vi "example_2_2010.vi"() -> ()   [LabVIEW 2010]
uses:
  <vilib>/Analysis/NI_AALBase.lvlib
  <vilib>/Analysis/baseanly.llb/Mean (DBL).vi
panel:
  out "Time with \"On\"":u32
  out "Time with \"Auto\"":u32
  in  "Time dimensions":bool
  out "MAE Theil-Sen (Off)":dbl format="%0.2f"
  out "MAE Theil-Sen (Auto)":dbl format="%0.2f"
  out "XY Graph":cluster{dbl[], dbl[]}[](graph)
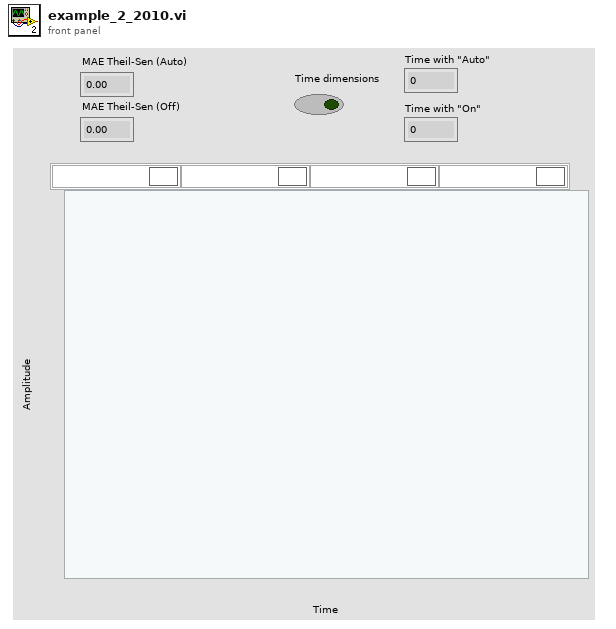
[diagram p1: front panel]
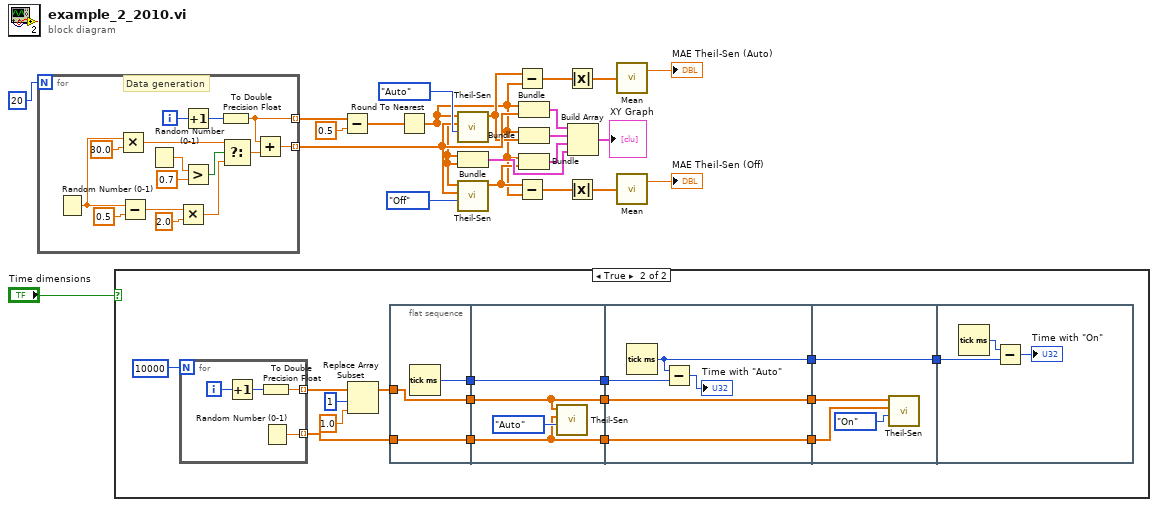
[diagram p0: block diagram]
diagram:
  n1 = for {
    N: 20 -> [_]
    tunnel: [w25] -> w14 mode=indexing
    tunnel: [w23] -> w17 mode=indexing
    i -> [w35]
    # "Data generation"
    n2 = Random Number (0-1)() -> (number: 0 to 1=w27:dbl)
    n3 = Multiply(x=w27, y=30.0 ("t")) -> (x*y=w26:dbl)
    n4 = Subtract(x=w27, y=0.5) -> (x-y=w37:dbl)
    n5 = Random Number (0-1)() -> (number: 0 to 1=w33:dbl)
    n6 = Multiply(x=w37, y=2.0) -> (x*y=w30:dbl)
    n7 = Increment(x=w35) -> (x+1=w34:i32)
    n8 = Greater?(x=w33, y=0.7) -> (0:w29:bool)
    n9 = To Double Precision Float(number=w34) -> (double precision float=w25:dbl)
    n10 = Select(t=w26, s=w29, f=w30) -> (s? t:f=w24:dbl)
    n11 = Add(x=w25, y=w24) -> (x+y=w23:dbl)
  }
  n12 = case shown="True" "Time dimensions" {
    frame False {
    }
    frame True {
      n13 = for {
        N: 10000 -> [_]
        tunnel: [w55] -> w51 mode=indexing
        tunnel: [w54] -> w41 mode=indexing
        i -> [w56]
        n14 = Increment(x=w56) -> (x+1=w57:i32)
        n15 = To Double Precision Float(number=w57) -> (double precision float=w54:dbl)
        n16 = Random Number (0-1)() -> (number: 0 to 1=w55:dbl)
      }
      n17 = Replace Array Subset(array=w41, new element=1.0 ("new element/subarray"), index=1) -> (w38:dbl[])
      n18 = flat-sequence {
        tunnel: [w60] -> w52
        tunnel: w51 -> [w60]
        tunnel: w38 -> [w59]
        tunnel: [w59] -> w50
        tunnel: [w58] -> w45
        tunnel: w52 -> [w62]
        tunnel: w50 -> [w63]
        tunnel: [w63] -> w48
        tunnel: [w62] -> w47
        tunnel: w45 -> [w61]
        tunnel: [w61] -> w44
        tunnel: [w69] -> w49
        tunnel: w48 -> [w69]
        tunnel: w47 -> [w68]
        tunnel: [w68] -> w46
        tunnel: w44 -> [w67]
        tunnel: [w65] -> w43
        tunnel: w49 -> [w72]
        tunnel: w46 -> [w71]
        tunnel: w43 -> [w70]
        tunnel: [w70] -> w42
        tunnel: w42 -> [w75]
        frame #0 {
          n19 = Tick Count (ms)() -> (millisecond timer value=w58:u32)
        }
        frame #1 {
          n20 = call "Theil-Sen.vi"("Sen parameter"=enum16{"Auto", "On", "Off"}."Auto", "input_Y"=w62, "input_X"=w63) -> ()  [unwired: 3 in, 4 out]
        }
        frame #2 {
          n21 = Tick Count (ms)() -> (millisecond timer value=w65:u32)
          n22 = Subtract(x=w65, y=w67) -> (x-y=→"Time with \"Auto\"":u32)
        }
        frame #3 {
          n23 = call "Theil-Sen.vi"("Sen parameter"=enum16{"Auto", "On", "Off"}."On", "input_Y"=w71, "input_X"=w72) -> ()  [unwired: 3 in, 4 out]
        }
        frame #4 {
          n24 = Tick Count (ms)() -> (millisecond timer value=w76:u32)
          n25 = Subtract(x=w76, y=w75) -> (x-y=→"Time with \"On\"":u32)
        }
      }
    }
  }
  n26 = Subtract(x=w14, y=0.5) -> (x-y=w12:dbl[])
  n27 = Round To Nearest(number=w12) -> (nearest integer value=w2:dbl[])
  n28 = call "Theil-Sen.vi"("Sen parameter"=enum16{"Auto", "On", "Off"}."Auto", "input_Y"=w17, "input_X"=w2) -> ("output_Y"=w10:dbl[])  [unwired: 3 in, 3 out]
  n29 = Bundle(w2, w2) -> (w19:cluster{dbl[], dbl[]})  [unwired: 1 in]
  n30 = call "Theil-Sen.vi"("Sen parameter"=enum16{"Auto", "On", "Off"}."Off", "input_Y"=w17, "input_X"=w2) -> ("output_Y"=w3:dbl[])  [unwired: 3 in, 3 out]
  n31 = Subtract(x=w10, y=w2) -> (x-y=w9:dbl[])
  n32 = Subtract(x=w3, y=w2) -> (x-y=w4:dbl[])
  n33 = Bundle(w2, w17) -> (w22:cluster{dbl[], dbl[]})  [unwired: 1 in]
  n34 = Bundle(w2, "output_Y"=w10) -> (w21:cluster{dbl[], "output_Y":dbl[]})  [unwired: 1 in]
  n35 = Bundle(w2, "output_Y"=w3) -> (w15:cluster{dbl[], "output_Y":dbl[]})  [unwired: 1 in]
  n36 = Absolute Value(x=w9) -> (abs(x)=w8:dbl[])
  n37 = Absolute Value(x=w4) -> (abs(x)=w5:dbl[])
  n38 = Build Array(w22, w21, w15, w19) -> (→"XY Graph":cluster{dbl[], "output_Y":dbl[]}[])
  n39 = call-poly <vilib>:"Mean.vi"("X"=w8) -> ("mean"=→"MAE Theil-Sen (Auto)":dbl)  [unwired: 1 out]
  n40 = call-poly <vilib>:"Mean.vi"("X"=w5) -> ("mean"=→"MAE Theil-Sen (Off)":dbl)  [unwired: 1 out]
